vi "Enqueue Message.vi"   [LabVIEW 2020, in "Message Queue.lvlib"]
doc: "Pour un message normal, placer le message à la fin de la file d'attente. Pour un message prioritaire, l'ajouter au début de la file."
uses:
  Message Queue.lvlib
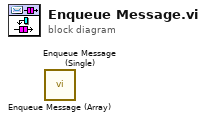
[diagram p0: block diagram]
diagram:
  n1 = call "Enqueue Message (Array).vi"() -> ()  [unwired: 10 in, 2 out]
  n2 = call "Enqueue Message (Single).vi"() -> ()  [unwired: 10 in, 2 out]
